vi "UserAccessFGV.vi"(7 "Enum":T1(ring), 8 "error in (no error)":errorcluster, 10 "User Name":string) -> (0 "error out":errorcluster, 2 "User Level":string)   [LabVIEW 2021]
uses:
  <vilib>/Utility/file.llb/Read Delimited Spreadsheet (string).vi
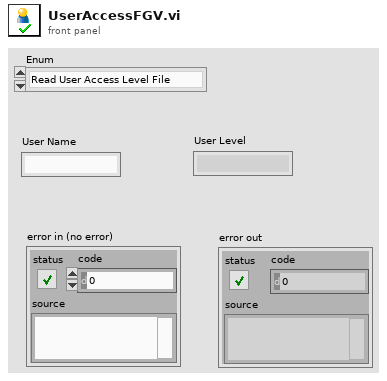
[diagram p1: front panel]
types:
  T1 = enum16{"Read User Access Level File", "Set Current User", "Get User Access Level"}
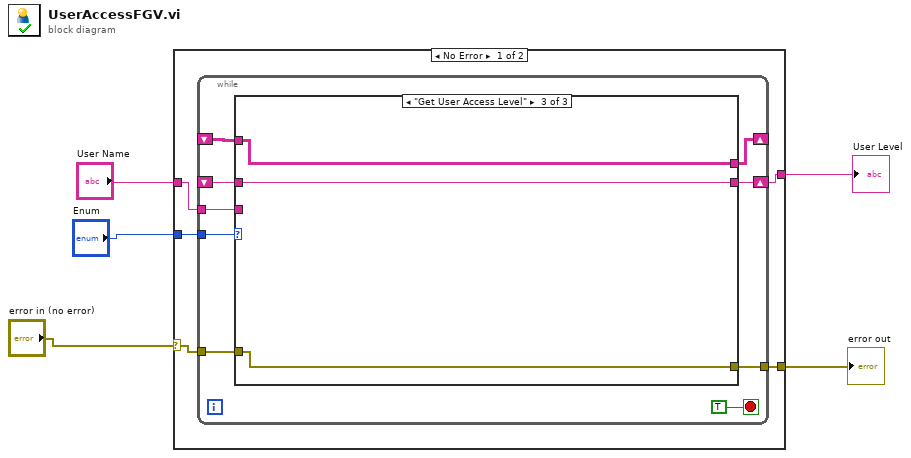
[diagram p0: block diagram]
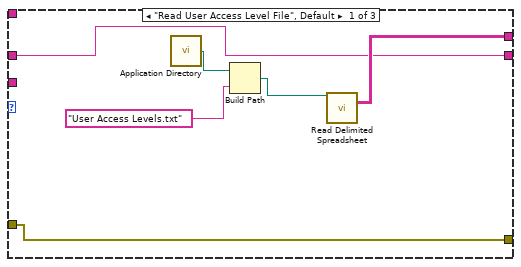
[diagram p2: hidden frame]
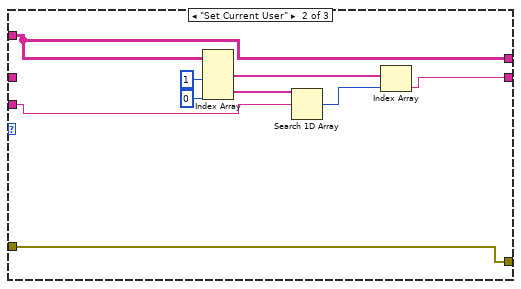
[diagram p3: hidden frame]
diagram:
  n1 = case shown="No Error" "error in (no error)" {
    selector: "error in (no error)" -> [w7 w38]
    tunnel: "Enum" -> [w10 _]
    tunnel: "User Name" -> [w6 w39]
    tunnel: [w9 w39] -> w2
    tunnel: [w8 w38] -> w1
    frame No Error {
      n2 = while {
        tunnel: w10 -> [w18]
        shift-right: [w17] -> _
        shift-left: _ -> [w16]
        shift-right: [w14] -> w9
        shift-left: _ -> [w15]
        tunnel: [w13] -> w8
        tunnel: w7 -> [w12]
        tunnel: w6 -> [w11]
        stop <- TRUE stop-if-true
        n3 = case shown="\"Get User Access Level\"" w18 {
          tunnel: [w22 w27 w37] -> w17
          tunnel: w16 -> [_ w27 w37]
          tunnel: w15 -> [w20 _ w36]
          tunnel: [w20 w29 w36] -> w14
          tunnel: [w21 w28 w35] -> w13
          tunnel: w12 -> [w21 w28 w35]
          tunnel: w11 -> [_ w26 _]
          frame "Read User Access Level File", Default {
            n4 = call <vilib>:"Application Directory.vi"() -> ("Application Directory"=w25:path)
            n5 = Build Path(base path=w25, name or relative path="User Access Levels.txt") -> (appended path=w23:path)
            n6 = call-poly <vilib>:"Read Delimited Spreadsheet.vi"("file path (dialog if empty)"=w23) -> ("all rows"=w22:string[][])  [unwired: 9 in, 5 out]
          }
          frame "Set Current User" {
            n7 = Index Array(array=w27, index (col) #1=1 ("disabled index (col)"), index (col) #2=0 ("index (col)")) -> (element #1=w31:string[], element #2=w32:string[])  [unwired: 2 in]
            n8 = Search 1D Array(1D array=w32, element=w26) -> (index of element=w30:i32)  [unwired: 1 in]
            n9 = Index Array(array=w31, index=w30) -> (element=w29:string)
          }
          frame "Get User Access Level" {
          }
        }
      }
    }
    frame Error {
    }
  }
  "error out" <- w1
  "User Level" <- w2
